vi "Get Manufacturer.vi"(8 "error in (no error)":errorcluster, 11 "Device in":refnum<class "Device.lvclass">) -> (0 "error out":errorcluster, 2 "Manufacturer":string, 3 "Device out":refnum<class "Device.lvclass">)   [LabVIEW 2021, in "RTL-SDR.lvlib" / "Device.lvclass"]
uses:
  Device.lvclass
  Device.lvclass/Device.ctl
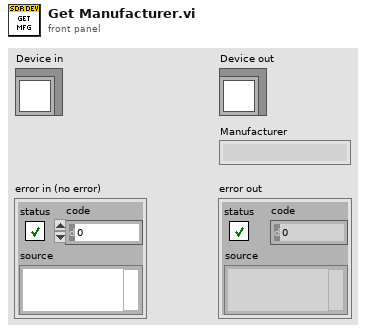
[diagram p1: front panel]
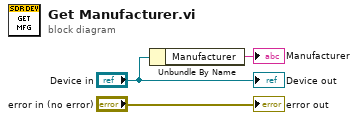
[diagram p0: block diagram]
diagram:
  n1 = Unbundle By Name("Device in") -> ("Manufacturer"=→"Manufacturer":string)
  "error out" <- "error in (no error)"
  "Device out" <- "Device in"
